vi "AI-Motor_Control.vi"(8 "Error In":errorcluster, 11 "目標位置(0~4095)":u16) -> (0 "Error Out":errorcluster)   [LabVIEW 2019]
uses:
  <instrlib>/Dynamixel Motor/Public/Motor Operation/Low Level/Baud Setting.ctl
  Variable/Position.vi
  <instrlib>/Dynamixel Motor/Dynamixel Motor.lvlib
panel:
  in  "Stop":bool
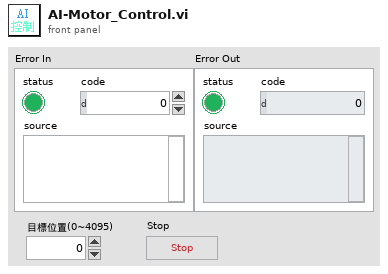
[diagram p1: front panel]
types:
  T1 = typedef "Dynamixel Motor.lvlib/Baud Setting.ctl" = u8
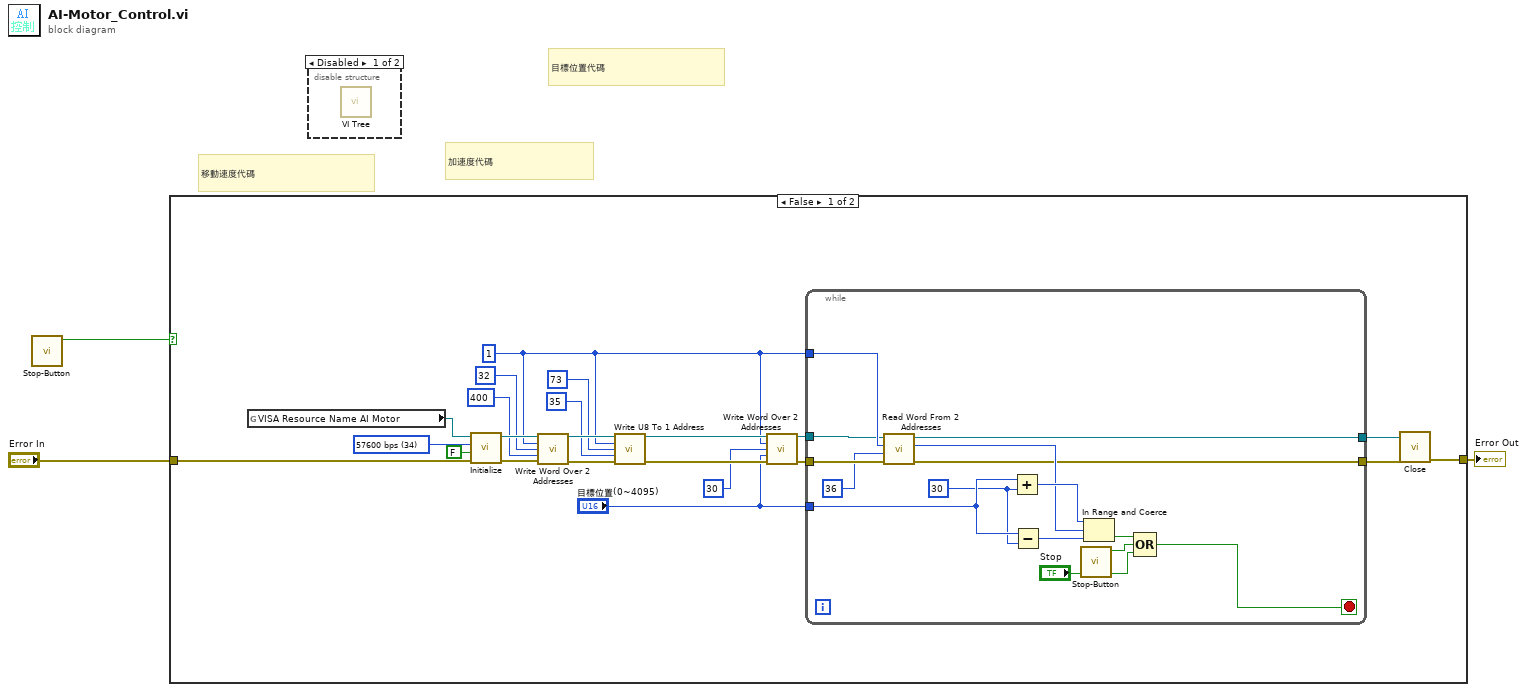
[diagram p0: block diagram]
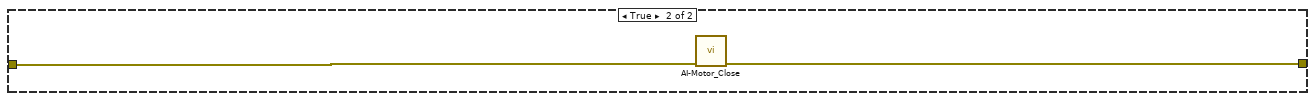
[diagram p2: hidden frame]
diagram:
  # "目標位置代碼"
  # "加速度代碼"
  # "移動速度代碼"
  n1 = call "Stop-Button.vi"() -> ("顯示按下?"=w1:bool)  [unwired: 10 in, 1 out]
  n2 = case shown="False" w1 {
    tunnel: "Error In" -> [w5 w42]
    tunnel: [w15 w41] -> w2
    frame False {
      w8 = u8 1 ("Motor ID (0)")
      w25 = T1 34 items=["1,000,000 bps"=1, "500,000 bps"=3, "400,000 bps"=4, "250,000 bps"=7, "200,000 bps"=9, "115200 bps"=16, "57600 bps"=34, "19200 bps"=103, "9600 bps"=207] ("Baud rate (57600 bps)")
      n3 = global read "Position.vi" "VISA Resource Name AI Motor"() -> (w4:refnum<visa-resource-name>)
      n4 = call <instrlib>:"Initialize.vi"("error in (no error)"=w5, "Force Baud Rate (True)"=FALSE, "Baud rate (57600 bps)"=w25, "VISA resource name"=w4) -> ("error out"=w23:errorcluster, "VISA resource name out"=w24:refnum<visa-resource-name>)  [unwired: 6 in]
      n5 = call <instrlib>:"Write Word Over 2 Addresses.vi"("VISA resource name"=w24, "Motor ID (0)"=w8, "Address number (0)"=u8 32, "Parameter (0)"=u16 400, "error in (no error)"=w23) -> ("VISA resource name out"=w20:refnum<visa-resource-name>, "error out"=w17:errorcluster)  [unwired: 9 in]
      n6 = call <instrlib>:"Write U8 To 1 Address.vi"("VISA resource name"=w20, "Motor ID (0)"=w8, "Address number (0)"=u8 73, "Parameter (0)"=u16 35, "error in (no error)"=w17) -> ("VISA resource name out"=w10:refnum<visa-resource-name>, "error out"=w11:errorcluster)  [unwired: 9 in]
      n7 = call <instrlib>:"Write Word Over 2 Addresses.vi"("VISA resource name"=w10, "Motor ID (0)"=w8, "Address number (0)"=u8 30 ("Motor ID (0)"), "Parameter (0)"="目標位置(0~4095)", "error in (no error)"=w11) -> ("VISA resource name out"=w6:refnum<visa-resource-name>, "error out"=w12:errorcluster)  [unwired: 9 in]
      n8 = while {
        tunnel: "目標位置(0~4095)" -> [w28]
        tunnel: w8 -> [w40]
        tunnel: w12 -> [w39]
        tunnel: [w30] -> w14
        tunnel: [w29] -> w13
        tunnel: w6 -> [w26]
        stop <- w31 stop-if-true
        w27 = u8 30 ("y")
        n9 = call <instrlib>:"Read Word From 2 Addresses.vi"("Error in (no error)"=w39, "Address number (0)"=u8 36, "Motor ID (0)"=w40, "VISA resource name"=w26) -> ("error out"=w30:errorcluster, "Data"=w34:u16, "VISA resource name out"=w29:refnum<visa-resource-name>)  [unwired: 5 in]
        n10 = Add(x=w28, y=w27) -> (x+y=w37:u16)
        n11 = Subtract(x=w28, y=w27) -> (x-y=w36:u16)
        n12 = call "Stop-Button.vi"() -> ("顯示按下?"=w33:bool)  [unwired: 10 in, 1 out]
        n13 = In Range and Coerce(upper limit=w37, x=w34, lower limit=w36) -> (In Range?=w35:bool)  [unwired: 1 out]
        n14 = Compound Arithmetic op=OR(w35, w33, "Stop") -> (w31:bool)
      }
      n15 = call <instrlib>:"Close.vi"("error in (no error)"=w14, "VISA resource name"=w13) -> ("error out"=w15:errorcluster)  [unwired: 9 in]
    }
    frame True {
      n16 = call "AI-Motor_Close.vi"("Error In"=w42) -> ("Error Out"=w41:errorcluster)  [unwired: 10 in]
    }
  }
  "Error Out" <- w2
  n17 = disable-structure shown="Disabled" {
    frame Disabled {
      n18 = call <instrlib>:"VI Tree.vi"() -> ()  [unwired: 12 in]
    }
    frame Enabled {
    }
  }
